vi "notify_event_listenters.vi"(8 "error in (no error)":errorcluster, 10 "Base Class (LabVIEW Object)":refnum<class>, 11 "Default Lookup in":refnum<class "Default Lookup.lvclass">) -> (0 "error out":errorcluster, 3 "Default Lookup out":refnum<class "Default Lookup.lvclass">)   [LabVIEW 2019, in "Default Lookup.lvclass"]
uses:
  Default Lookup.lvclass
  Default Lookup.lvclass/Default Lookup.ctl
  LVCOOOP.lvlib
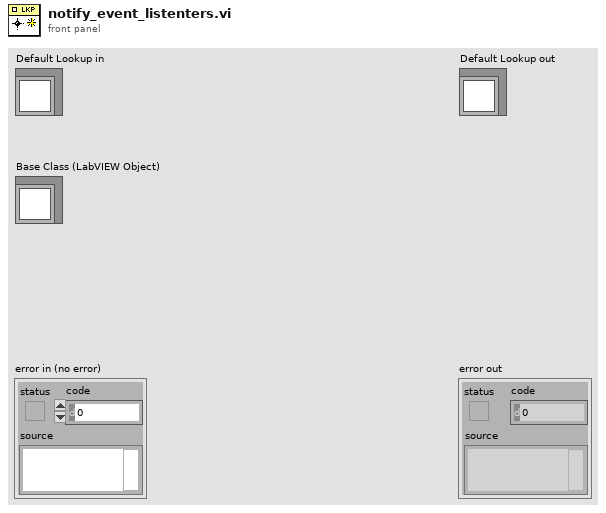
[diagram p1: front panel]
types:
  T1 = typedef "Default Lookup.lvclass/lookup_data.ctl" = cluster{"instances":refnum<data-value>[], "listeners":refnum<user-event>[]}
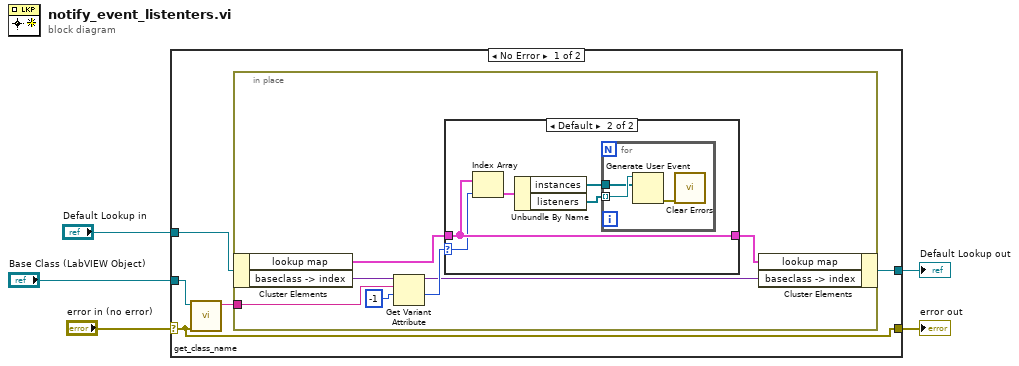
[diagram p0: block diagram]
diagram:
  n1 = case shown="No Error" "error in (no error)" {
    selector: "error in (no error)" -> [w9 w28]
    tunnel: [w9 w28] -> w4
    tunnel: [w6 w27] -> w2
    tunnel: "Default Lookup in" -> [w8 w27]
    tunnel: "Base Class (LabVIEW Object)" -> [w10 _]
    frame No Error {
      n2 = call "get_class_name.vi"("error in (no error)"=w9, "LabVIEW Object in"=w10) -> ("class name"=w7:string)  [unwired: 8 in, 1 out]
      n3 = in-place {
        in-place-border: w7 -> [w16]
        n4 = in-place-cluster #1(w8) -> ("lookup map"=w12:T1[], "baseclass -> index"=w17:variant)
        n5 = Get Variant Attribute(Variant=w17, name=w16, default value (empty Variant)=-1) -> (duplicate Variant=w11:variant, value=w14:i32)  [unwired: 1 in, 2 out]
        n6 = case shown="Default" w14 {
          selector: w14 -> [_ w22]
          tunnel: [w18 w23] -> w13
          tunnel: w12 -> [w18 w23]
          frame -1 {
          }
          frame Default {
            n7 = Index Array(array=w23, index=w22) -> (element=w21:T1)
            n8 = Unbundle By Name(w21) -> ("instances"=w19:refnum<data-value>[], "listeners"=w20:refnum<user-event>[])
            n9 = for {
              tunnel: w20 -> [w26] mode=indexing
              tunnel: w19 -> [w25]
              n10 = Generate User Event(user event=w26, event data cluster=w25) -> (error out=w24:errorcluster)  [unwired: 2 in, 1 out]
              n11 = call "Clear Errors.vi"("error in (no error)"=w24) -> ()  [unwired: 10 in, 1 out]
            }
          }
        }
        n12 = in-place-cluster #1("lookup map"=w13, "baseclass -> index"=w11) -> (w6:refnum<class "Default Lookup.lvclass">)
      }
    }
    frame Error {
    }
  }
  "error out" <- w4
  "Default Lookup out" <- w2
